vi "_DAC Calibration.vi"(2 "DAC in":string[][](table), 3 "Board":T1 items=["Quad DC Board", "Lens 1 (Slot 8) Module", "Lens 2 (Slot 6) Module", "Detector Board", "Quad DC Board with Test Points", "Lens 1 Module with Test Points", "Len 2 Module with Test Points", "", "", "", "", ""]) -> (0 "aborted":bool, 1 "DAC out":string[][](table))   [LabVIEW 2012]
uses:
  Type/_Board ID.ctl
  Type/_RT Active Ch.ctl
  Configuration/_Global Configuration.vi
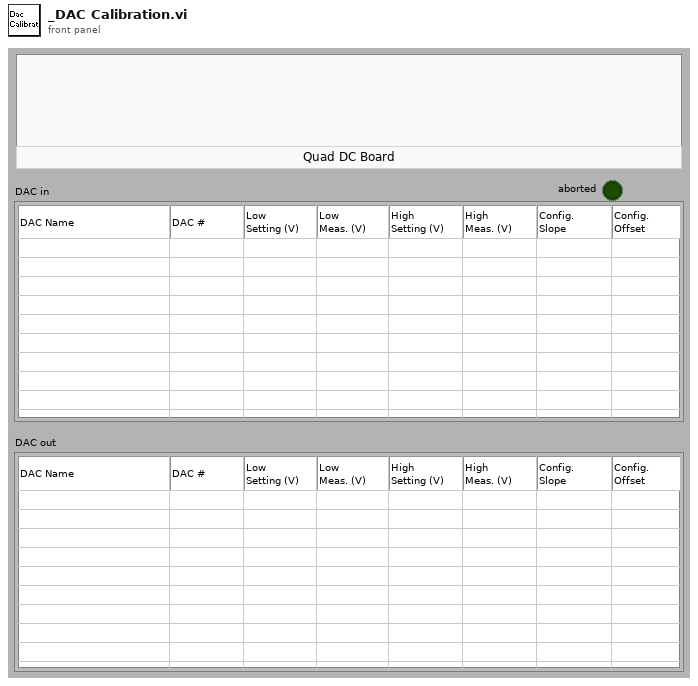
[diagram p1: front panel]
types:
  T1 = typedef "_Board ID.ctl" = u16
  T2 = typedef "_RT Configuration 2.ctl" = cluster{"Name":string, "Ch#":u8, "Min":dbl, "Max":dbl, "Def+":dbl, "Def-":dbl, "Offset":dbl, "Slope":dbl, "Type":u8, "Description":string, "SettleT":dbl}
  T3 = typedef "_RT Active Ch.ctl" = cluster{"Start":i32, "Step":i32, "ChID":i32}
  T4 = typedef "_RT Instrument 2.ctl" = cluster{"Table":T2[], "Instrument":string[]}
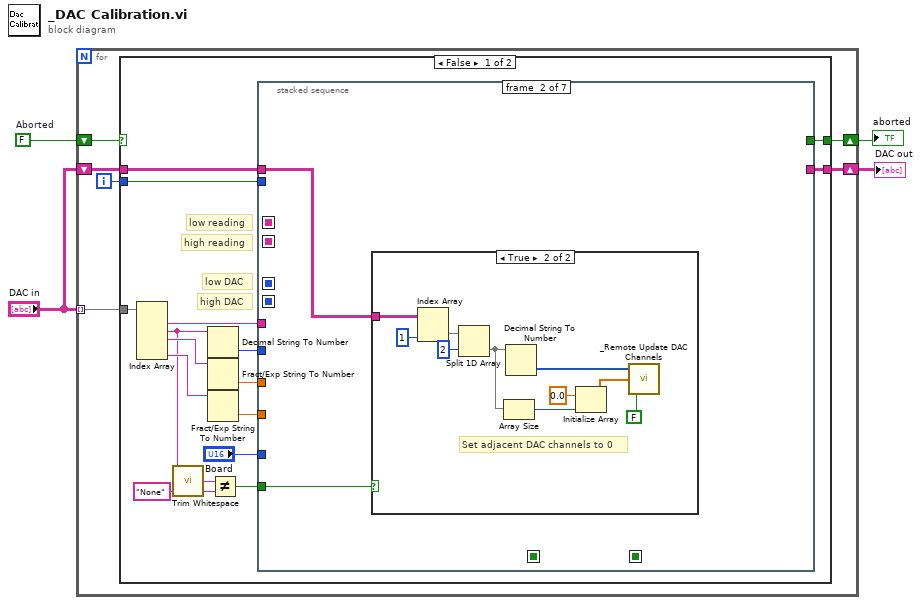
[diagram p0: block diagram]
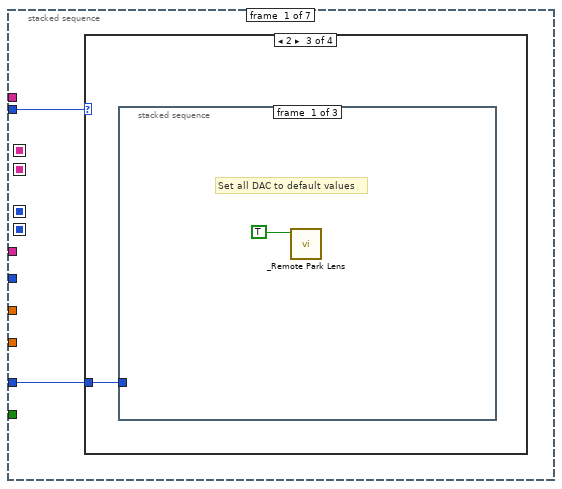
[diagram p2: hidden frame]
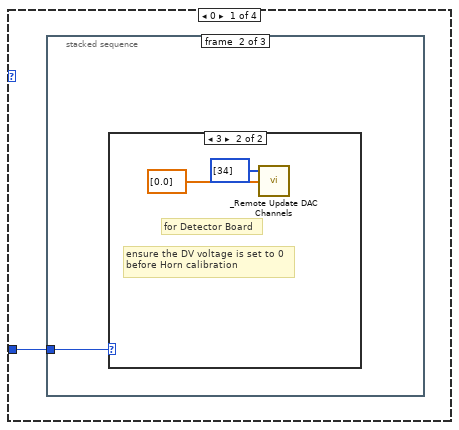
[diagram p3: hidden frame]
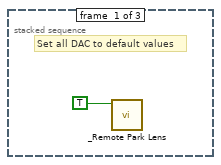
[diagram p4: hidden frame]
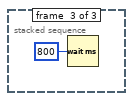
[diagram p6: hidden frame]
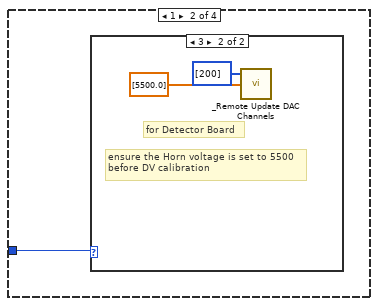
[diagram p7: hidden frame]
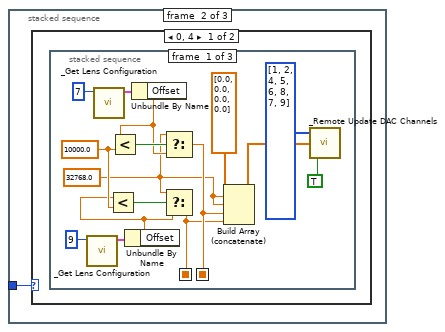
[diagram p9: hidden frame]
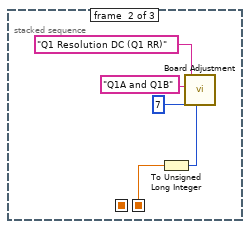
[diagram p10: hidden frame]
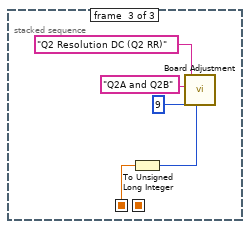
[diagram p11: hidden frame]
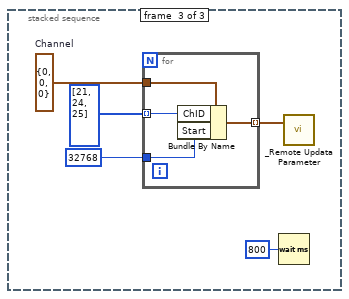
[diagram p13: hidden frame]
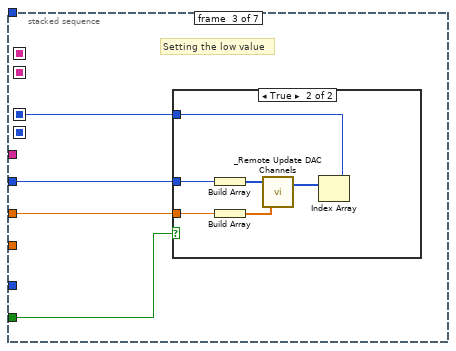
[diagram p16: hidden frame]
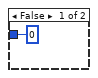
[diagram p17: hidden frame]
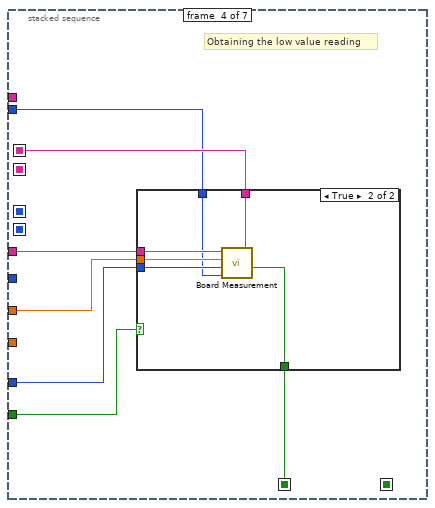
[diagram p18: hidden frame]
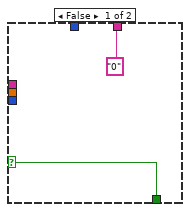
[diagram p19: hidden frame]
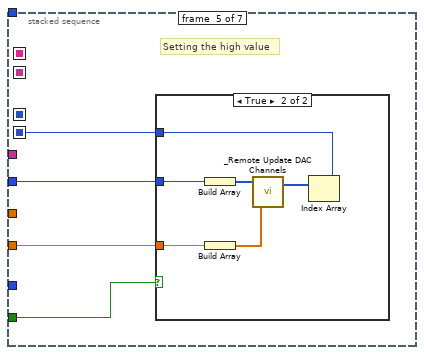
[diagram p20: hidden frame]
diagram:
  w2 = FALSE  # Aborted
  n1 = for {
    tunnel: "DAC in" -> [w10] mode=indexing
    shift-right: [w7] -> w3
    shift-left: "DAC in" -> [w8]
    shift-right: [w5] -> w1
    shift-left: w2 -> [w6]
    i -> [w9]
    n2 = case shown="False" w6 {
      selector: w6 -> [_ w195]
      tunnel: w10 -> [w26 _]
      tunnel: w9 -> [w23 _]
      tunnel: w8 -> [w19 w194]
      tunnel: [w17 w194] -> w7
      tunnel: [w11 w195] -> w5
      frame False {
        # "high DAC"
        # "low DAC"
        # "high reading"
        # "low reading"
        n3 = Index Array(array=w26) -> (element #1=w16:string, element #2=w12:string, element #3=w25:string, element #5=w20:string)  [unwired: 5 in, 1 out]
        n4 = call <vilib>:"Trim Whitespace.vi"("string"=w12) -> ("trimmed string"=w14:string)  [unwired: 1 in]
        n5 = Decimal String To Number(string=w12) -> (number=w24:i32)  [unwired: 3 out]
        n6 = Fract/Exp String To Number(string=w25) -> (number=w22:dbl)  [unwired: 4 out]
        n7 = Fract/Exp String To Number(string=w20) -> (number=w21:dbl)  [unwired: 4 out]
        n8 = Not Equal?(x=w14, y="None") -> (x != y?=w13:bool)
        n9 = stacked-sequence {
          seq-local: [_ _ w89 _ _ _ _] -> [_ _ _ _ _ _ w149]
          seq-local: [_ _ _ _ w116 _ _] -> [_ _ _ _ _ _ w150]
          seq-local: [_ _ _ w102 _ _ _] -> [_ _ _ _ _ _ w145]
          seq-local: [_ _ _ _ _ w129 _] -> [_ _ _ _ _ _ w144]
          seq-local: [_ _ _ w99 _ _ _] -> [_ _ _ _ _ w126 _]
          seq-local: [_ _ _ _ _ w125 _] -> [_ _ _ _ _ _ w141]
          tunnel: w24 -> [_ _ w91 _ w117 _ w143]
          tunnel: w23 -> [w28 _ _ w101 _ w127 w146]
          tunnel: w22 -> [_ _ w90 w104 _ _ _]
          tunnel: w21 -> [_ _ _ _ w115 w128 _]
          tunnel: w16 -> [_ _ _ w105 _ w131 _]
          tunnel: w19 -> [_ w76 _ _ _ _ w147]
          tunnel: "Board" -> [w27 _ _ w103 _ w130 w140]
          tunnel: [_ _ _ _ _ _ w148] -> w17
          tunnel: w13 -> [_ w77 w88 w100 w114 _ w142]
          tunnel: [_ _ _ _ _ w125 _] -> w11
          frame #0 {
            n10 = case shown="2" w28 {
              tunnel: w27 -> [w29 w35 w38 _]
              frame 0 {
                n11 = stacked-sequence {
                  tunnel: w29 -> [_ w31 _]
                  frame #0 {
                    # "Set all DAC to default values"
                    n12 = call "_Remote Park Lens.vi"("All Ch (F)"=TRUE) -> ()  [unwired: 1 in, 6 out]
                  }
                  frame #1 {
                    n13 = case shown="3" w31 {
                      frame 0, Default {
                      }
                      frame 3 {
                        # "ensure the DV voltage is set to 0\nbefore Horn calibration"
                        # "for Detector Board"
                        n14 = call "_Remote Update DAC Channels.vi"("UserValue"=dbl[] [0.0], "Ch#"=i32[] [34]) -> ()  [unwired: 1 in, 2 out]
                      }
                    }
                  }
                  frame #2 {
                    n15 = Wait (ms)(milliseconds to wait=u32 800) -> ()  [unwired: 1 out]
                  }
                }
              }
              frame 1 {
                n16 = case shown="3" w35 {
                  frame 0, Default {
                  }
                  frame 3 {
                    # "ensure the Horn voltage is set to 5500\nbefore DV calibration"
                    # "for Detector Board"
                    n17 = call "_Remote Update DAC Channels.vi"("UserValue"=dbl[] [5500.0], "Ch#"=i32[] [200]) -> ()  [unwired: 1 in, 2 out]
                  }
                }
              }
              frame 2 {
                n18 = stacked-sequence {
                  tunnel: w38 -> [_ w40 _]
                  frame #0 {
                    # "Set all DAC to default values"
                    n19 = call "_Remote Park Lens.vi"("All Ch (F)"=TRUE) -> ()  [unwired: 1 in, 6 out]
                  }
                  frame #1 {
                    n20 = case shown="0, 4" w40 {
                      frame 0, 4 {
                        n21 = stacked-sequence {
                          seq-local: [w43 _ _] -> [_ _ w63]
                          seq-local: [w44 _ _] -> [_ w58 _]
                          frame #0 {
                            w41 = 32768.0 ("y")
                            w47 = 10000.0 ("y")
                            n22 = call "_Get Lens Configuration.vi"("Channel #"=u8 9) -> ("Lens Configuration"=w52:T2)  [unwired: 1 in, 5 out]
                            n23 = call "_Get Lens Configuration.vi"("Channel #"=u8 7) -> ("Lens Configuration"=w53:T2)  [unwired: 1 in, 5 out]
                            n24 = Unbundle By Name(w52) -> ("Offset"=w46:dbl)
                            n25 = Less?(x=w46, y=w47) -> (x < y?=w48:bool)
                            n26 = Unbundle By Name(w53) -> ("Offset"=w49:dbl)
                            n27 = Less?(x=w49, y=w47) -> (x < y?=w50:bool)
                            n28 = Select(t=w41, s=w50, f=w49) -> (s? t:f=w44:dbl)
                            n29 = Select(t=w41, s=w48, f=w46) -> (s? t:f=w43:dbl)
                            n30 = Build Array (concatenate)(dbl[] [0.0, 0.0, 0.0, 0.0] ("Ch#"), w41, w41, w44, w43) -> (w45:dbl[])
                            n31 = call "_Remote Update DAC Channels.vi"("In DAC(F)"=TRUE ("Zero-DAC (F)"), "UserValue"=w45, "Ch#"=u8[] [1, 2, 4, 5, 6, 8, 7, 9]) -> ()  [unwired: 2 out]
                          }
                          frame #1 {
                            n32 = To Unsigned Long Integer(number=w58) -> (unsigned 32bit integer=w57:u32)
                            n33 = call "Board Adjustment.vi"("DAC Value"=w57, "DAC Ch#"=7, "Test Points"="Q1A and Q1B" ("Expected Outcome"), "DAC Channel Name"="Q1 Resolution DC (Q1 RR)") -> ()  [unwired: 1 in, 4 out]
                          }
                          frame #2 {
                            n34 = To Unsigned Long Integer(number=w63) -> (unsigned 32bit integer=w62:u32)
                            n35 = call "Board Adjustment.vi"("DAC Value"=w62, "DAC Ch#"=9, "Test Points"="Q2A and Q2B" ("Expected Outcome"), "DAC Channel Name"="Q2 Resolution DC (Q2 RR)") -> ()  [unwired: 1 in, 4 out]
                          }
                        }
                      }
                      frame 1, Default {
                      }
                    }
                  }
                  frame #2 {
                    w68 = T3 {"Start"=0, "Step"=0, "ChID"=0}  # Channel
                    n36 = for {
                      tunnel: u8[] [21, 24, 25] ("Ch#") -> [w75] mode=indexing
                      tunnel: 32768 ("Start") -> [w74]
                      tunnel: w68 -> [w73]
                      tunnel: [w72] -> w67 mode=indexing
                      n37 = Bundle By Name(cluster=w73, "ChID"=w75, "Start"=w74) -> (w72:T3)
                    }
                    n38 = Wait (ms)(milliseconds to wait=u32 800) -> ()  [unwired: 1 out]
                    n39 = call "_Remote Updata Parameter.vi"("Parameters"=w67) -> ()  [unwired: 1 in, 1 out]
                  }
                }
              }
              frame Default {
              }
            }
          }
          frame #1 {
            n40 = case shown="True" w77 {
              tunnel: w76 -> [_ w78]
              frame False {
              }
              frame True {
                # "Set adjacent DAC channels to 0"
                n41 = Index Array(array=w78, index (col)=1 ("disabled index (col)")) -> (element=w86:string[])  [unwired: 1 in]
                n42 = Split 1D Array(array=w86, index=2) -> (second subarray=w84:string[])  [unwired: 1 out]
                n43 = Array Size(array=w84) -> (size(s)=w83:i32)
                n44 = Decimal String To Number(string=w84) -> (number=w80:i32[])  [unwired: 3 out]
                n45 = Initialize Array(0.0 ("element"), w83) -> (w79:dbl[])
                n46 = call "_Remote Update DAC Channels.vi"("In DAC(F)"=FALSE ("Zero-DAC (F)"), "UserValue"=w79, "Ch#"=w80) -> ()  [unwired: 2 out]
              }
            }
          }
          frame #2 {
            # "Setting the low value"
            n47 = case shown="True" w88 {
              tunnel: w91 -> [_ w98]
              tunnel: w90 -> [_ w96]
              tunnel: [0 ("Channel #") w93] -> w89
              frame False {
              }
              frame True {
                n48 = Build Array(w98) -> (w97:i32[])
                n49 = Build Array(w96) -> (w95:dbl[])
                n50 = call "_Remote Update DAC Channels.vi"("UserValue"=w95, "Ch#"=w97) -> ("DACValue"=w94:i32[])  [unwired: 1 in, 1 out]
                n51 = Index Array(array=w94) -> (element=w93:i32)  [unwired: 1 in]
              }
            }
          }
          frame #3 {
            # "Obtaining the low value reading"
            n52 = case shown="True" w100 {
              selector: w100 -> [w106 _]
              tunnel: w105 -> [_ w113]
              tunnel: w104 -> [_ w112]
              tunnel: w103 -> [_ w111]
              tunnel: ["0" w110] -> w102
              tunnel: w101 -> [_ w109]
              tunnel: [w106 w108] -> w99
              frame False {
              }
              frame True {
                n53 = call "Board Measurement.vi"("index"=w109, "Board"=w111, "Expected Reading"=w112, "DAC Channel Name"=w113) -> ("Aborted"=w108:bool, "Reading"=w110:string)  [unwired: 2 out]
              }
            }
          }
          frame #4 {
            # "Setting the high value"
            n54 = case shown="True" w114 {
              tunnel: w117 -> [_ w124]
              tunnel: [-5900 ("Channel #") w120] -> w116
              tunnel: w115 -> [_ w119]
              frame False {
              }
              frame True {
                n55 = Build Array(w124) -> (w123:i32[])
                n56 = Build Array(w119) -> (w122:dbl[])
                n57 = call "_Remote Update DAC Channels.vi"("UserValue"=w122, "Ch#"=w123) -> ("DACValue"=w121:i32[])  [unwired: 1 in, 1 out]
                n58 = Index Array(array=w121) -> (element=w120:i32)  [unwired: 1 in]
              }
            }
          }
          frame #5 {
            # "Obtaining the high value reading"
            n59 = case shown="False" w126 {
              selector: w126 -> [_ w139]
              tunnel: w131 -> [w137 _]
              tunnel: w130 -> [w136 _]
              tunnel: [w135 ""] -> w129
              tunnel: w128 -> [w134 _]
              tunnel: w127 -> [w133 _]
              tunnel: [w132 w139] -> w125
              frame False {
                n60 = call "Board Measurement.vi"("index"=w133, "Board"=w136, "Expected Reading"=w134, "DAC Channel Name"=w137) -> ("Aborted"=w132:bool, "Reading"=w135:string)  [unwired: 2 out]
              }
              frame True {
              }
            }
          }
          frame #6 {
            n61 = case shown="False" w141 {
              tunnel: w150 -> [w174 _]
              tunnel: w149 -> [w173 _]
              tunnel: [w165 w193] -> w148
              tunnel: w147 -> [w161 w193]
              tunnel: w146 -> [w152 _]
              tunnel: w145 -> [w159 _]
              tunnel: w144 -> [w158 _]
              tunnel: w143 -> [w157 _]
              tunnel: w142 -> [w156 _]
              tunnel: w140 -> [w155 _]
              frame False {
                w171 = i16 4 ("precision (6)")
                # "Slope"
                # "-b"
                # "offset"
                # "m"
                # "D2-D1"
                # "R2-R1"
                n62 = Fract/Exp String To Number(string=w158) -> (number=w181:dbl)  [unwired: 4 out]
                n63 = Fract/Exp String To Number(string=w159) -> (number=w177:dbl)  [unwired: 1 in, 3 out]
                n64 = Replace Array Subset(array=w161, new element=w159, index (row)=w152, index (col)=3 ("disabled index (col)")) -> (w164:string[][])
                n65 = Subtract(x=w181, y=w177) -> (x-y=w180:dbl)
                n66 = Subtract(x=w174, y=w173) -> (x-y=w179:i32)
                n67 = Replace Array Subset(array=w164, new element=w158, index (row)=w152, index (col)=5 ("disabled index (col)")) -> (w160:string[][])
                n68 = Divide(x=w180, y=w179) -> (x/y=w175:dbl)
                n69 = Reciprocal(x=w175) -> (1/x=w172:dbl)
                n70 = Multiply(x=w175, y=w173) -> (x*y=w178:dbl)
                n71 = Subtract(x=w178, y=w177) -> (x-y=w176:dbl)
                n72 = Divide(x=w176, y=w175) -> (x/y=w154:dbl)
                n73 = call "_Check Offset.vi"("Board"=w155, "Row#"=w152, "Offset In"=w154) -> ("Offset Out"=w153:dbl)
                n74 = case shown="True" w156 {
                  tunnel: w172 -> [_ w189]
                  tunnel: w157 -> [_ w187]
                  tunnel: w153 -> [w182 w183]
                  tunnel: [w182 w183] -> w151
                  frame False {
                  }
                  frame True {
                    n75 = call "_Get Lens Configuration.vi"("Channel #"=w187) -> ("Config Row#"=w191:i32)  [unwired: 1 in, 5 out]
                    n76 = global read "_Global Configuration.vi" "Configuration 2"() -> (w185:T4)
                    n77 = Unbundle By Name(w185) -> ("Table"=w188:T2[])
                    n78 = Index Array(array=w188, index=w191) -> (element=w192:T2)
                    n79 = Bundle By Name(cluster=w192, "Offset"=w183, "Slope"=w189) -> (w190:T2)
                    n80 = Replace Array Subset(array=w188, new element=w190, index=w191) -> (w186:T2[])
                    n81 = Bundle By Name(cluster=w185, "Table"=w186) -> (w184:T4)
                    n82 = global write "_Global Configuration.vi" "Configuration 2"(w184) -> ()
                  }
                }
                n83 = Number To Fractional String(number=w172, precision (6)=w171) -> (F-format string=w169:string)  [unwired: 2 out]
                n84 = Number To Fractional String(number=w151, precision (6)=w171) -> (F-format string=w166:string)  [unwired: 2 out]
                n85 = Replace Array Subset(array=w160, new element=w169, index (row)=w152, index (col)=6 ("disabled index (col)")) -> (w167:string[][])
                n86 = Replace Array Subset(array=w167, new element=w166, index (row)=w152, index (col)=7 ("disabled index (col)")) -> (w165:string[][])
              }
              frame True {
              }
            }
          }
        }
      }
      frame True {
      }
    }
  }
  "DAC out" <- w3
  "aborted" <- w1
